vi "多参数标样核查对话框.vi"() -> (2 "确认":bool, 3 "输出参数":T1)   [LabVIEW 2016, in "斯坦道原位多参数.lvlib"]
panel:
  in  "浊度":bool
  in  "电导率":bool
  in  "pH":bool
  in  "DO":bool
  in  "水温":bool
  in  "取消":bool
  in  "确定":bool
  # "请输入启动参数"
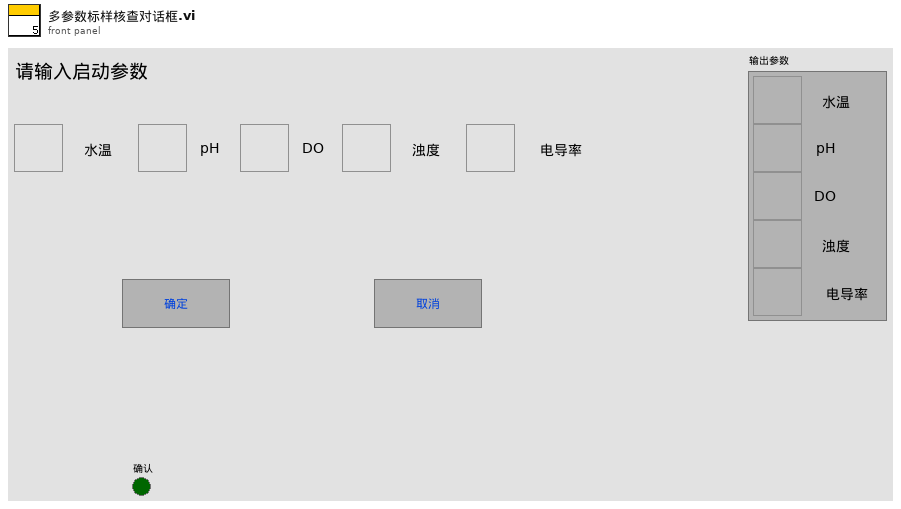
[diagram p1: front panel]
types:
  T1 = cluster{"水温":bool, "pH":bool, "DO":bool, "浊度":bool, "电导率":bool}
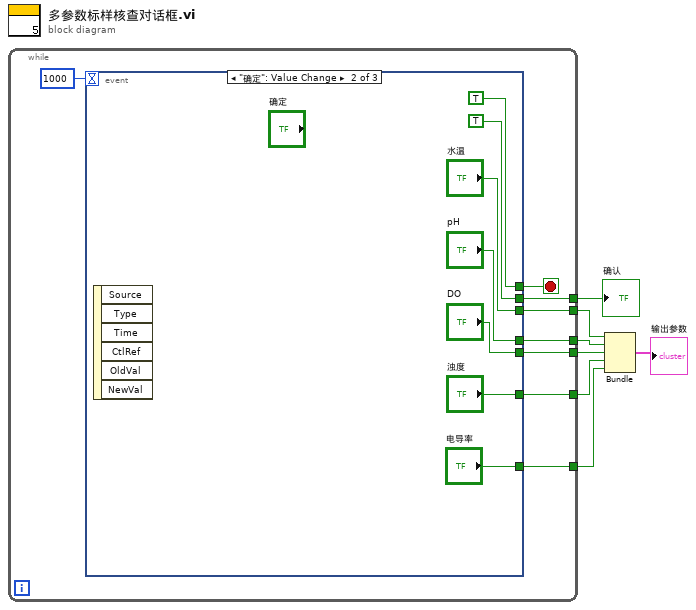
[diagram p0: block diagram]
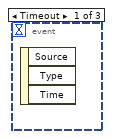
[diagram p2: hidden frame]
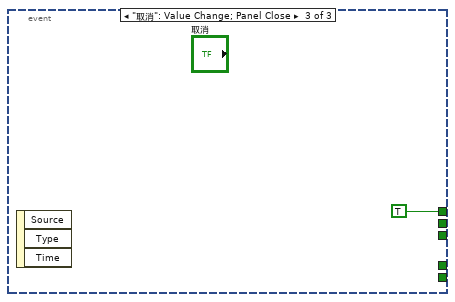
[diagram p3: hidden frame]
diagram:
  n1 = while {
    tunnel: [w13] -> w7
    tunnel: [w12] -> w6
    tunnel: [w11] -> w5
    tunnel: [w10] -> w1
    tunnel: [w9] -> w2
    tunnel: [w8] -> w4
    stop <- w15 stop-if-true
    n2 = event shown="[1] \"确定\": Value Change" {
      selector: _ -> [_ _ _]
      dyn-events: _ -> [_ _ _]
      timeout: 1000 -> [_ _ _]
      tunnel: [_ TRUE TRUE] -> w15
      tunnel: [_ TRUE _] -> w13
      tunnel: [_ "水温" _] -> w12
      tunnel: [_ "pH" _] -> w11
      tunnel: [_ "电导率" _] -> w10
      tunnel: [_ "浊度" _] -> w9
      tunnel: [_ "DO" _] -> w8
      event Timeout {
        n3 = event-data() -> ()  [unwired: 1 in, 3 out]
      }
      event "确定": Value Change {
        n4 = event-data() -> ()  [unwired: 1 in, 6 out]
      }
      event "取消": Value Change; Panel Close {
        n5 = event-data() -> ()  [unwired: 1 in, 3 out]
      }
    }
  }
  "确认" <- w7
  n6 = Bundle("水温"=w6, "pH"=w5, "DO"=w4, "浊度"=w2, "电导率"=w1) -> (→"输出参数":T1)  [unwired: 1 in]
